vi "Lookup_Table.vi"(0 "Y_Array":dbl[](array[numeric]) format="%.2f", 1 "x_in":dbl, 2 "X_Array":dbl[](array[numeric]) format="%.2f") -> (6 "y_out":dbl format="%.2f")   [LabVIEW 2018, in "ArgosLib.lvlib"]
uses:
  ArgosLib.lvlib
panel:
  # "Lookup_Table"
  # "This subsystem is a lookup table and will linerly interolate between points in the array"
  # "Tunning"
  # "Inputs"
  # "Outputs"
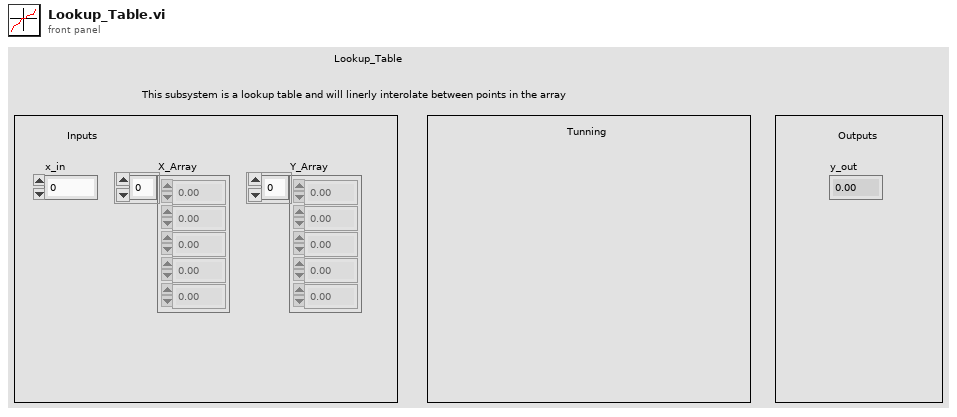
[diagram p1: front panel]
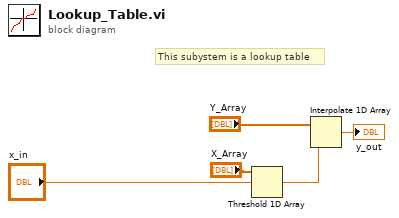
[diagram p0: block diagram]
diagram:
  # "This subystem is a lookup table"
  n1 = Threshold 1D Array(2:"x_in", 3:"X_Array") -> (0:w1:dbl)  [unwired: 1 in]
  n2 = Interpolate 1D Array(1:w1, 2:"Y_Array") -> (0:→"y_out":dbl)
